vi "Check version ini.vi"(7 "Alert user on version update (F)":bool, 8 "error in":errorcluster, 10 "Version String":string="Version", 11 "refnum in":T1) -> (0 "error out":errorcluster, 3 "refnum":T1, 6 "Version changed":bool)   [LabVIEW 2013, in "FileIO lib.lvlib"]
doc: "Reads the [APPLICATION] Version. key and overwrites it with the incomming verison string. Alerts the user if the version has changed."
uses:
  FileIO lib.lvlib
  <vilib>/Utility/config.llb/Config Data RefNum.ctl
  <vilib>/Utility/config.llb/Read Key (String).vi
  <vilib>/Utility/config.llb/Write Key (String).vi
  <vilib>/Utility/config.llb/NI_LVConfig.lvlib
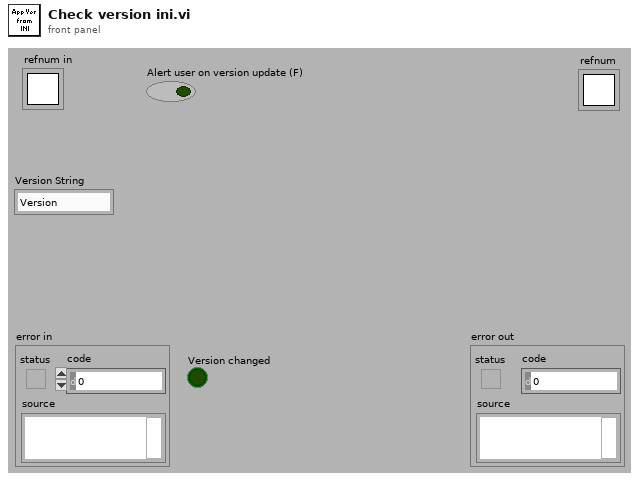
[diagram p1: front panel]
types:
  T1 = typedef "NI_LVConfig.lvlib/Config Data RefNum.ctl" = refnum<k1>
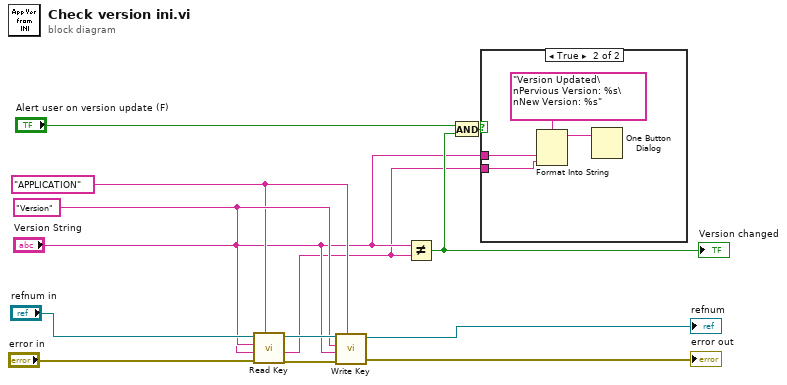
[diagram p0: block diagram]
diagram:
  w6 = "APPLICATION" ("key")
  w9 = "Version" ("key")
  n1 = call-poly <vilib>:"Read Key.vi"("section"=w6, "error in (no error)"="error in", "default value"="Version String", "key"=w9, "refnum"="refnum in") -> ("error out"=w10:errorcluster, "value"=w1:string, "refnum out"=w11:T1)  [unwired: 3 in, 1 out]
  n2 = call-poly <vilib>:"Write Key.vi"("section"=w6, "error in (no error)"=w10, "value"="Version String", "key"=w9, "refnum"=w11) -> ("error out"=→"error out":errorcluster, "refnum out"=→"refnum":T1)  [unwired: 4 in, 1 out]
  n3 = Not Equal?(x="Version String", y=w1) -> (x != y?=w5:bool)
  "Version changed" <- w5
  n4 = And(x="Alert user on version update (F)", y=w5) -> (x .and. y?=w3:bool)
  n5 = case shown="True" w3 {
    tunnel: "Version String" -> [_ w17]
    tunnel: w1 -> [_ w16]
    frame False {
    }
    frame True {
      n6 = Format Into String(format string="Version Updated\nPervious Version: %s\nNew Version: %s", w17, w16) -> (resulting string=w14:string)  [unwired: 2 in, 1 out]
      n7 = One Button Dialog(message=w14) -> ()  [unwired: 1 in, 1 out]
    }
  }
